vi "Configure Marker Search.vi"(0 "VISA resource name":refnum<visa-resource-name>, 1 "Peak Polarity (0: Positive)":u16(ring) items=["Positive", "Negative", "Both"], 2 "Peak Excursion (3.0)":dbl=3.0 format="%^.2e", 3 "Target Value (0.0)":dbl format="%^.2e", 4 "Target Polarity (0: Positive)":u16(ring) items=["Positive", "Negative", "Both"], 5 "error in (no error)":errorcluster, 6 "Channel (1)":i32=1, 7 "Partial Marker State (F: Disable)":bool, 8 "Marker (1)":i32=1, 9 "Start Value (0.0)":dbl format="%^.2e", 10 "Range Coupling (F: Disable)":bool, 11 "Stop Value (0.0)":dbl format="%^.2e", 12 "Tracking (F: Disable)":bool) -> (14 "VISA resource name out":refnum<visa-resource-name>, 19 "error out":errorcluster)   [LabVIEW 2020, in "Agilent ENA Series.lvlib"]
doc: "Configures the marker search."
uses:
  <instrlib>/Agilent ENA Series/Agilent ENA Series.lvlib
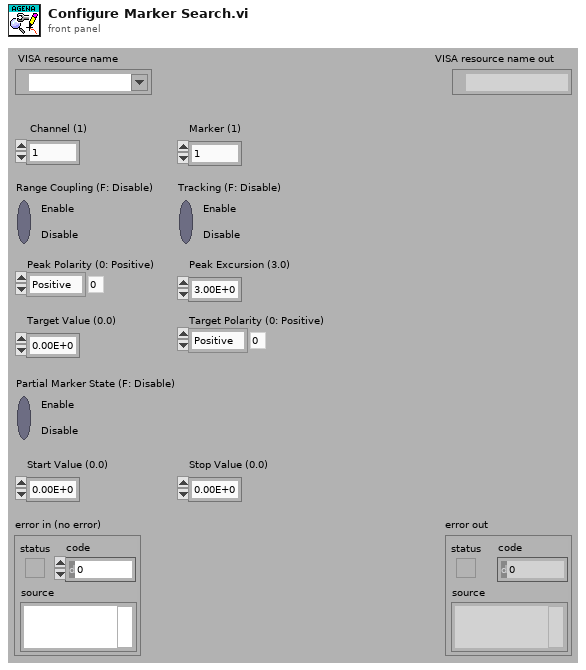
[diagram p1: front panel]
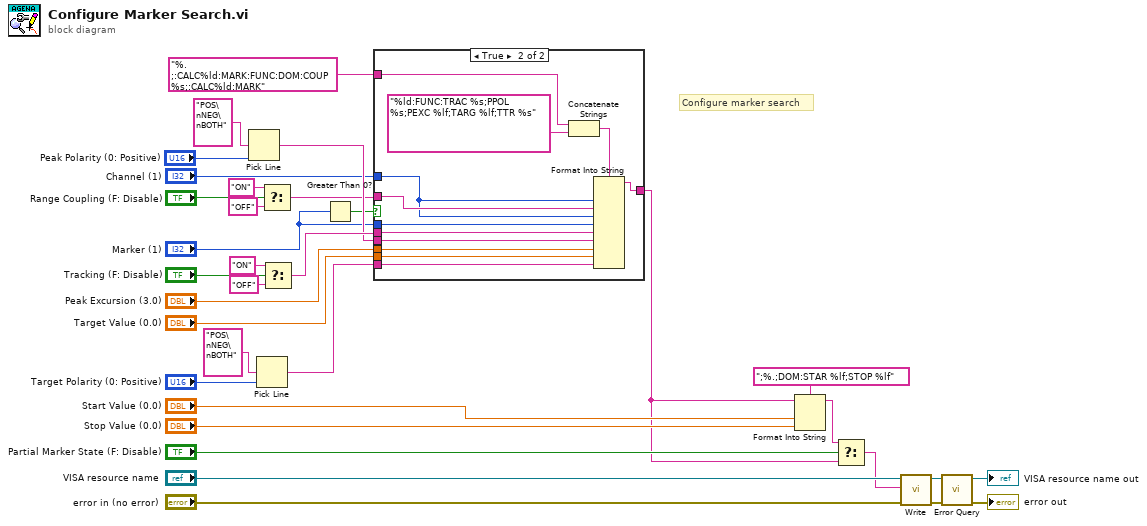
[diagram p0: block diagram]
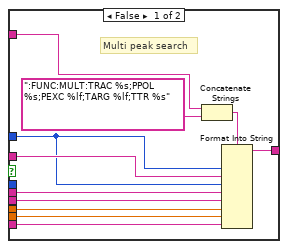
[diagram p2: hidden frame]
diagram:
  # "Configure marker search"
  n1 = Pick Line(multi-line string="POS\nNEG\nBOTH", line index="Peak Polarity (0: Positive)") -> (output string=w22:string)  [unwired: 1 in]
  n2 = Pick Line(multi-line string="POS\nNEG\nBOTH", line index="Target Polarity (0: Positive)") -> (output string=w17:string)  [unwired: 1 in]
  n3 = Select(t="ON", s="Range Coupling (F: Disable)", f="OFF") -> (s? t:f=w1:string)
  n4 = Select(t="ON", s="Tracking (F: Disable)", f="OFF") -> (s? t:f=w25:string)
  n5 = Greater Than 0?(x="Marker (1)") -> (x > 0?=w2:bool)
  n6 = case shown="True" w2 {
    tunnel: w1 -> [w42 w56]
    tunnel: w25 -> [w41 w55]
    tunnel: w22 -> [w40 w54]
    tunnel: "Peak Excursion (3.0)" -> [w39 w53]
    tunnel: "Target Value (0.0)" -> [w38 w52]
    tunnel: w17 -> [w37 w51]
    tunnel: "Channel (1)" -> [w34 w45]
    tunnel: [w35 w50] -> w6
    tunnel: "%.;:CALC%ld:MARK:FUNC:DOM:COUP %s;:CALC%ld:MARK" ("format string") -> [w36 w48]
    tunnel: "Marker (1)" -> [_ w46]
    frame False {
      # "Multi peak search"
      n7 = Concatenate Strings(w36, ":FUNC:MULT:TRAC %s;PPOL %s;PEXC %lf;TARG %lf;TTR %s" ("format string")) -> (w43:string)
      n8 = Format Into String(format string=w43, w34, w42, w34, w41, w40, w39, w38, w37) -> (resulting string=w35:string)  [unwired: 2 in, 1 out]
    }
    frame True {
      n9 = Concatenate Strings(w48, "%ld:FUNC:TRAC %s;PPOL %s;PEXC %lf;TARG %lf;TTR %s" ("format string")) -> (w47:string)
      n10 = Format Into String(format string=w47, w45, w56, w45, w46, w55, w54, w53, w52, w51) -> (resulting string=w50:string)  [unwired: 2 in, 1 out]
    }
  }
  n11 = Format Into String(format string=";%.;DOM:STAR %lf;STOP %lf", initial string=w6, "Start Value (0.0)", "Stop Value (0.0)") -> (resulting string=w7:string)  [unwired: 1 in, 1 out]
  n12 = Select(t=w7, s="Partial Marker State (F: Disable)", f=w6) -> (s? t:f=w5:string)
  n13 = call <instrlib>:"Write.vi"("error in (no error)"="error in (no error)", "String ()"=w5, "VISA resource name"="VISA resource name") -> ("error out"=w15:errorcluster, "VISA resource name out"=w16:refnum<visa-resource-name>)  [unwired: 6 in, 1 out]
  n14 = call <instrlib>:"Error Query.vi"("error in (no error)"=w15, "VISA resource name"=w16) -> ("error out"=→"error out":errorcluster, "VISA resource name out"=→"VISA resource name out":refnum<visa-resource-name>)  [unwired: 6 in, 2 out]
